vi "SDG60RefClock2(doesnt work).vi"(2 "error in (no error)":errorcluster, 3 "Ref 10MHz Src (T: Int)":bool=TRUE, 4 "10MHz Out (T:Enable)":bool=TRUE, 5 "VISA resource name":refnum<visa-resource-name>="USB0::0xF4EC::0x1101::SDG6XEBC5R0119::INSTR") -> (0 "error out":errorcluster, 1 "VISA resource name out":refnum<visa-resource-name>)   [LabVIEW 2018]
doc: "Configures the output impedance and source impedance for the channel you specify."
panel:
  # "If no valid external clock present,\noutputs will be switched off"
  # "Default state output state of\n10 MHz is off."
  # "Doesn't work!"
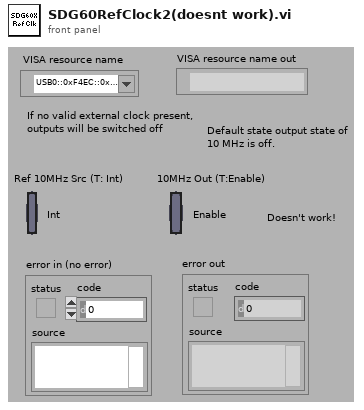
[diagram p1: front panel]
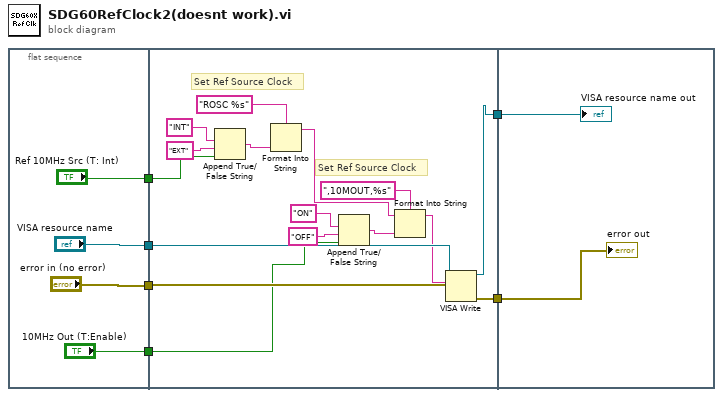
[diagram p0: block diagram]
diagram:
  n1 = flat-sequence {
    tunnel: ["Ref 10MHz Src (T: Int)"] -> w6
    tunnel: ["error in (no error)"] -> w5
    tunnel: ["VISA resource name"] -> w4
    tunnel: ["10MHz Out (T:Enable)"] -> w3
    tunnel: w6 -> [w22]
    tunnel: w5 -> [w21]
    tunnel: w4 -> [w20]
    tunnel: w3 -> [w14]
    tunnel: [w12] -> w2
    tunnel: [w11] -> w1
    tunnel: w2 -> [w28]
    tunnel: w1 -> [w27]
    frame #0 {
    }
    frame #1 {
      # "Set Ref Source Clock"
      # "Set Ref Source Clock"
      n2 = Append True/False String(1:w22, 2:"EXT" ("true string"), 3:"INT" ("true string")) -> (0:w23:string)  [unwired: 1 in]
      n3 = Format Into String(format string="ROSC %s", w23) -> (resulting string=w15:string)  [unwired: 2 in, 1 out]
      n4 = Append True/False String(1:w14, 2:"OFF" ("true string"), 3:"ON" ("true string")) -> (0:w16:string)  [unwired: 1 in]
      n5 = Format Into String(format string=",10MOUT,%s", initial string=w15, w16) -> (resulting string=w13:string)  [unwired: 1 in, 1 out]
      n6 = VISA Write(VISA resource name=w20, write buffer=w13, error in (no error)=w21) -> (VISA resource name out=w12:refnum<visa-resource-name>, error out=w11:errorcluster)  [unwired: 1 out]
    }
    frame #2 {
      "error out" <- w27
      "VISA resource name out" <- w28
    }
  }
